vi "Load Layout.vi"(8 "error in (no error)":errorcluster, 10 "Data":path, 11 "TabCtl":refnum<vi>[](array[refnum])) -> (0 "error out":errorcluster)   [LabVIEW 2020, in "MDI ViewManager.lvlib"]
uses:
  MDI ViewManager.lvlib
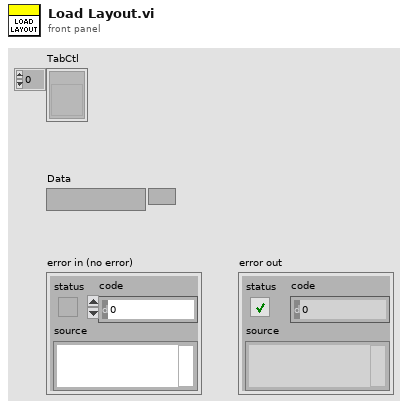
[diagram p1: front panel]
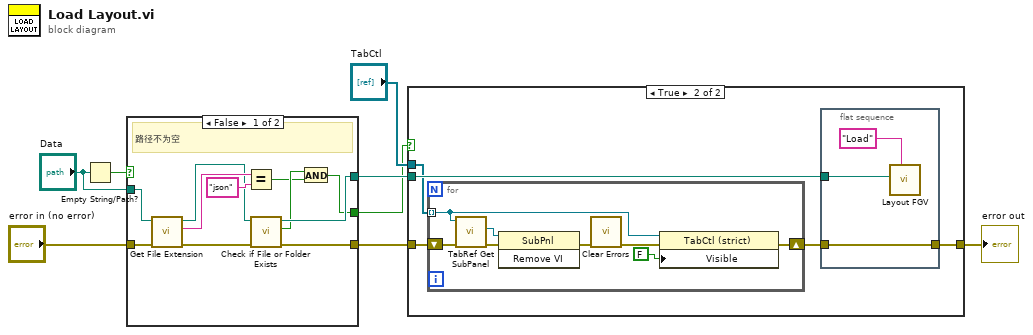
[diagram p0: block diagram]
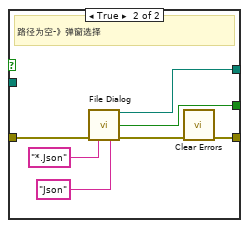
[diagram p3: hidden frame]
diagram:
  n1 = Empty String/Path?(string/path="Data") -> (empty?=w3:bool)
  n2 = case shown="False" w3 {
    tunnel: [w9 w26] -> w1
    tunnel: [w18 w25] -> w2
    tunnel: [w19 w21] -> w7
    tunnel: "error in (no error)" -> [w13 w20]
    tunnel: "Data" -> [w17 _]
    frame False {
      # "路径不为空"
      n3 = call <vilib>:"Get File Extension.vi"("error in (no error)"=w13, "file"=w17) -> ("error out"=w12:errorcluster, "lowercase file extension"=w16:string, "dup file"=w14:path)  [unwired: 5 in, 2 out]
      n4 = Equal?(x=w16, y="json") -> (x = y?=w10:bool)
      n5 = call <vilib>:"Check if File or Folder Exists.vi"("error in (no error)"=w12, "path"=w14) -> ("error out"=w19:errorcluster, "file or folder exists?"=w11:bool, "dup path"=w18:path)  [unwired: 7 in]
      n6 = And(x=w11, y=w10) -> (x .and. y?=w9:bool)
    }
    frame True {
      # "路径为空-》弹窗选择"
      n7 = call "File Dialog"("error in"=w20, "pattern (all files)"="*.Json", "pattern label"="Json") -> ("selected path"=w25:path, "exists"=w26:bool, "error out"=w24:errorcluster)  [unwired: 9 in, 1 out]
      n8 = call <vilib>:"Clear Errors.vi"("error in (no error)"=w24) -> ("error out"=w21:errorcluster)  [unwired: 5 in, 1 out]
    }
  }
  n9 = case shown="True" w1 {
    tunnel: w2 -> [_ w32]
    tunnel: "TabCtl" -> [_ w31]
    tunnel: w7 -> [w27 w30]
    tunnel: [w27 w28] -> w6
    frame False {
    }
    frame True {
      n10 = for {
        tunnel: w31 -> [w39] mode=indexing
        shift-right: [w36] -> w29
        shift-left: w30 -> [w37]
        n11 = call "TabRef Get SubPanel.vi"("error in (no error)"=w37, "TabControl in"=w39) -> ("error out"=w38:errorcluster, "Sub Panel"=w40:refnum<vi>)  [unwired: 7 in, 1 out]
        n12 = invoke class="SubPnl" method="Remove VI"(reference=w40, error in=w38) -> (error out=w42:errorcluster)  [unwired: 1 in, 2 out]
        n13 = call <vilib>:"Clear Errors.vi"("error in (no error)"=w42) -> ("error out"=w41:errorcluster)  [unwired: 5 in, 1 out]
        n14 = property class="TabCtl (strict)"(reference=w39, error in=w41, "Visible"=FALSE) -> (error out=w36:errorcluster)  [unwired: 1 out]
      }
      n15 = flat-sequence {
        tunnel: w32 -> [w35]
        tunnel: w29 -> [w34]
        tunnel: [w34] -> w28
        frame #0 {
          n16 = call "Layout FGV.vi"("String"="Load", "file (use dialog)"=w35) -> ()  [unwired: 10 in]
        }
      }
    }
  }
  "error out" <- w6
